vi "System Error Cluster Replacement.vi"(8 "error in (no error)":errorcluster, 11 "Folder Path":path) -> (0 "error out":errorcluster)   [LabVIEW 2017]
uses:
  <vilib>/Utility/traverseref.llb/TRef TravTarget.ctl
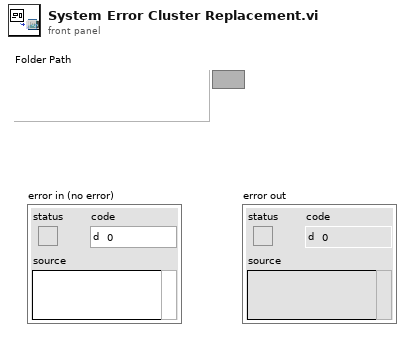
[diagram p1: front panel]
types:
  T1 = typedef "TRef TravTarget.ctl" = enum16{"FP", "BD", "Other"}
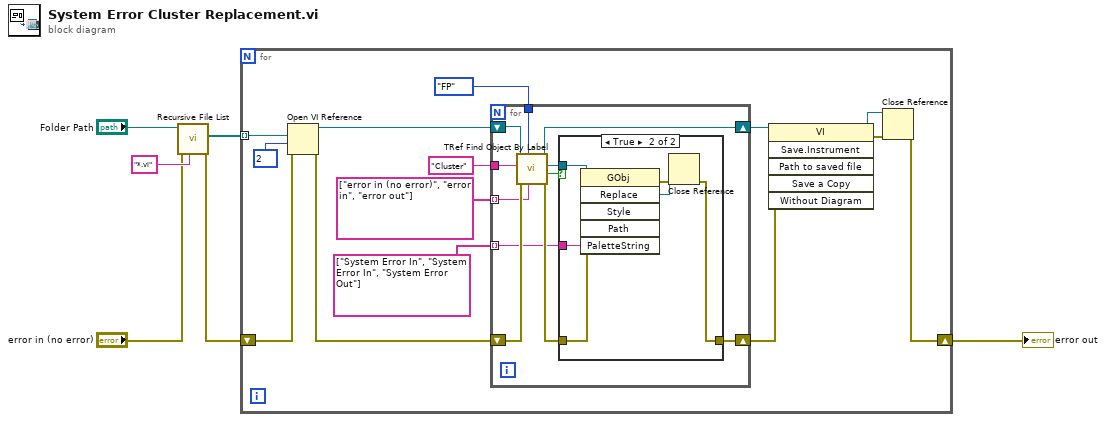
[diagram p0: block diagram]
diagram:
  n1 = call <vilib>:"Recursive File List.vi"("pattern"="*.vi", "error in (no error)"="error in (no error)", "Folder Path"="Folder Path") -> ("error out"=w1:errorcluster, "All Files in Dir"=w3:path[])  [unwired: 4 in, 3 out]
  n2 = for {
    shift-right: [w12] -> w6
    shift-left: w1 -> [w9]
    tunnel: w3 -> [w10] mode=indexing
    n3 = Open VI Reference(vi path=w10, options=2, error in (no error)=w9) -> (vi reference=w11:refnum<vi>, error out=w8:errorcluster)  [unwired: 3 in]
    n4 = for {
      tunnel: TRef_TravTarget."FP" ("Traverse Target") -> [w30]
      tunnel: "Cluster" ("Class Name") -> [w29]
      shift-right: [w26] -> w16
      shift-left: w11 -> [w31]
      tunnel: string[] ["error in (no error)", "error in", "error out"] -> [w22] mode=indexing
      tunnel: string[] ["System Error In", "System Error In", "System Error Out"] -> [w21] mode=indexing
      shift-right: [w25] -> w15
      shift-left: w8 -> [w23]
      n5 = call <vilib>:"TRef Find Object By Label.vi"("Label"=w22, "Traverse Target"=w30, "error in (no error)"=w23, "Class Name"=w29, "VI Ref"=w31) -> ("error out"=w27:errorcluster, "Found?"=w24:bool, "Found Obj Ref"=w28:refnum<vi>, "dup VI Ref"=w26:refnum<vi>)  [unwired: 3 in]
      n6 = case shown="True" w24 {
        tunnel: w28 -> [_ w38]
        tunnel: w27 -> [w32 w37]
        tunnel: w21 -> [_ w36]
        tunnel: [w32 w34] -> w25
        frame False {
        }
        frame True {
          n7 = invoke class="GObj" method="Replace"(reference=w38, error in=w37, "PaletteString"=w36) -> (error out=w35:errorcluster, "Replace"=w33:refnum<vi>)  [unwired: 3 in, 4 out]
          n8 = Close Reference(reference=w33, error in (no error)=w35) -> (error out=w34:errorcluster)
        }
      }
    }
    n9 = invoke class="VI" method="Save.Instrument"(reference=w16, error in=w15) -> (reference out=w14:refnum<vi>, error out=w13:errorcluster)  [unwired: 4 in, 4 out]
    n10 = Close Reference(reference=w14, error in (no error)=w13) -> (error out=w12:errorcluster)
  }
  "error out" <- w6
